vi "PowerRamp.vi"(11 "input cluster":T1) -> (0 "y right R":dbl, 1 "x right R":dbl, 2 "y left R":dbl, 3 "x left R":dbl)   [LabVIEW 2015]
uses:
  Joystick/ControlsToCommands.ctl
  <vilib>/ptbypt/NI_PtbyPt.lvlib
panel:
  in  "Low Pass Filter Average Length":dbl=0.05
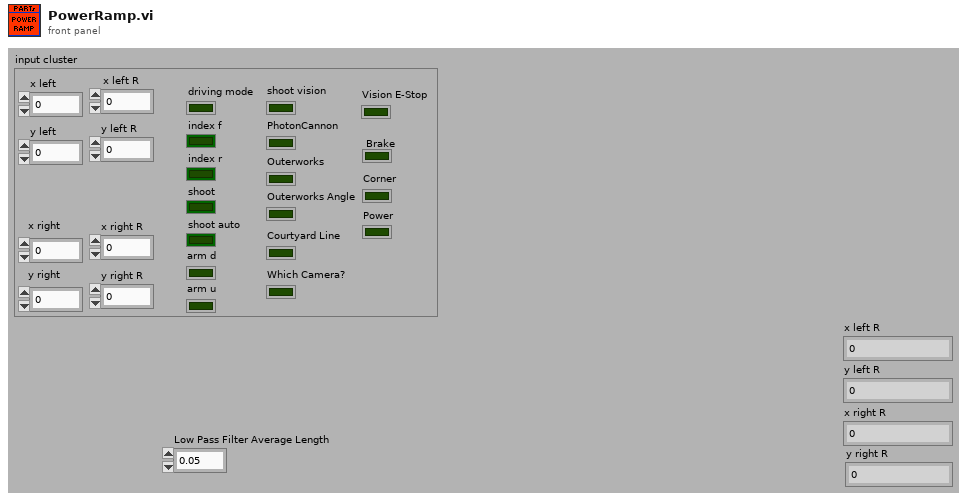
[diagram p1: front panel]
types:
  T1 = typedef "ControlsToCommands.ctl" = cluster{"x left":dbl, "y left":dbl, "x right":dbl, "y right":dbl, "driving mode":bool, "index f":bool, "index r":bool, "shoot":bool, "shoot auto":bool, "arm d":bool, "arm u":bool, "shoot vision":bool, "PhotonCannon":bool, "Outerworks":bool, "Outerworks Angle":bool, "Courtyard Line":bool, "Which Camera?":bool, "Vision E-Stop":bool, "x left R":dbl, "y left R":dbl, "x right R":dbl, "y right R":dbl, "Brake":bool, "Corner":bool, "Power":bool}
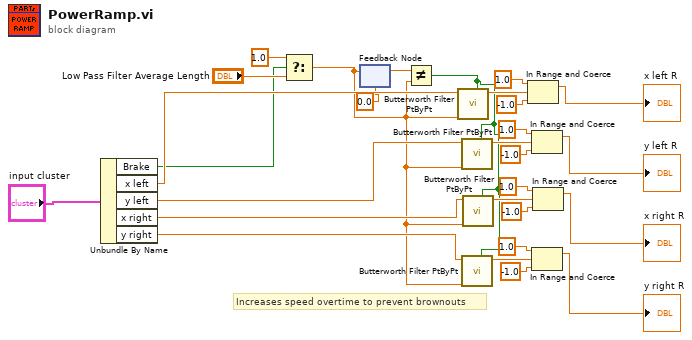
[diagram p0: block diagram]
diagram:
  # "Increases speed overtime to prevent brownouts"
  n1 = Unbundle By Name("input cluster") -> ("Brake"=w1:bool, "x left"=w14:dbl, "y left"=w13:dbl, "x right"=w12:dbl, "y right"=w11:dbl)
  n2 = Select(t=1.0, s=w1, f="Low Pass Filter Average Length") -> (s? t:f=w2:dbl)
  n3 = feedback #1(0.0 ("Low Pass Filter Average Length")) -> (w25:dbl)
  n4 = feedback-in #1(w2) -> ()
  n5 = Not Equal?(x=w25, y=w2) -> (x != y?=w15:bool)
  n6 = call <vilib>:"Butterworth Filter PtByPt.vi"("initialize"=w15, "low cutoff freq: fl"=w2, "x"=w14) -> ("Filtered x"=w28:dbl)  [unwired: 6 in, 1 out]
  n7 = call <vilib>:"Butterworth Filter PtByPt.vi"("initialize"=w15, "low cutoff freq: fl"=w2, "x"=w13) -> ("Filtered x"=w22:dbl)  [unwired: 6 in, 1 out]
  n8 = call <vilib>:"Butterworth Filter PtByPt.vi"("initialize"=w15, "low cutoff freq: fl"=w2, "x"=w11) -> ("Filtered x"=w16:dbl)  [unwired: 6 in, 1 out]
  n9 = call <vilib>:"Butterworth Filter PtByPt.vi"("initialize"=w15, "low cutoff freq: fl"=w2, "x"=w12) -> ("Filtered x"=w21:dbl)  [unwired: 6 in, 1 out]
  n10 = In Range and Coerce(upper limit=1.0, x=w28, lower limit=-1.0) -> (coerced(x)=→"x left R":dbl)  [unwired: 1 out]
  n11 = In Range and Coerce(upper limit=1.0, x=w22, lower limit=-1.0) -> (coerced(x)=→"y left R":dbl)  [unwired: 1 out]
  n12 = In Range and Coerce(upper limit=1.0, x=w16, lower limit=-1.0) -> (coerced(x)=→"y right R":dbl)  [unwired: 1 out]
  n13 = In Range and Coerce(upper limit=1.0, x=w21, lower limit=-1.0) -> (coerced(x)=→"x right R":dbl)  [unwired: 1 out]
